vi "readRegister.vi"(2 "Register to Read":u16, 3 "SPI Config In":T1) -> (0 "Register Data Out":u8[](array[numeric]), 1 "SPI Config Out":T1)   [LabVIEW 2019]
uses:
  SPI/SPI Config.ctl
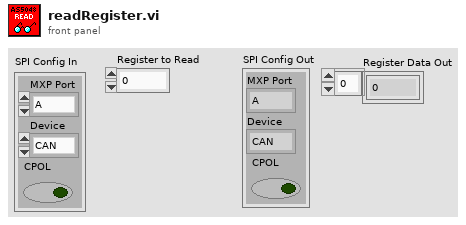
[diagram p1: front panel]
types:
  T1 = typedef "SPI Config.ctl" = cluster{"MXP Port":enum16{"A", "B"}, "Device":enum16{"CAN", "ENC", "IMU1", "IMU2"}, "CPOL":bool}
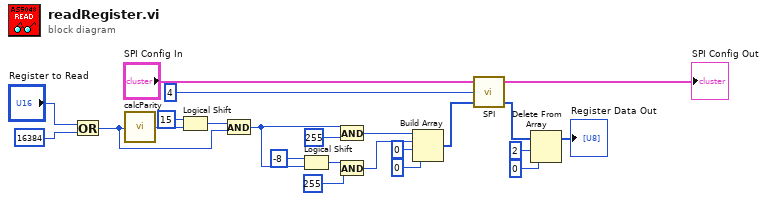
[diagram p0: block diagram]
diagram:
  n1 = Or(x="Register to Read", y=u16 16384) -> (x .or. y?=w16:u16)
  n2 = call "calcParity.vi"("Number"=w16) -> ("Parity"=w19:u16)
  n3 = Logical Shift(y=i16 15, x=w19) -> (x << y=w17:u16)
  n4 = And(x=w17, y=w16) -> (x .and. y?=w8:u16)
  n5 = Logical Shift(y=i16 -8, x=w8) -> (x << y=w12:u16)
  n6 = And(x=w8, y=u16 255) -> (x .and. y?=w14:u16)
  n7 = And(x=w12, y=u16 255) -> (x .and. y?=w10:u16)
  n8 = Build Array(w14, w10, u16 0 ("element"), u16 0 ("element")) -> (w13:u16[])
  n9 = call "SPI.vi"("Data to Write"=w13, "Frames to Write"=u8 4, "SPI Config In"="SPI Config In") -> ("Data Read"=w4:u8[], "SPI Config Out"=→"SPI Config Out":T1)  [unwired: 1 out]
  n10 = Delete From Array(array=w4, length=2, index=0) -> (array with subset deleted=→"Register Data Out":u8[])  [unwired: 1 out]
